vi "fric_comp_subvi.vi"(4 "Cpos":dbl, 5 "Cneg":dbl, 6 "Vpos":dbl, 7 "Vneg":dbl, 11 "Velocity":dbl) -> (3 "Numeric":dbl)   [LabVIEW 2018]
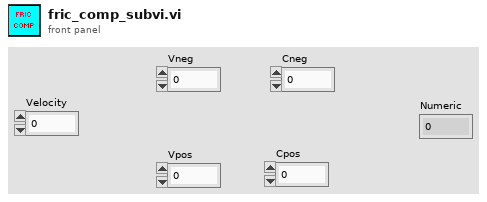
[diagram p1: front panel]
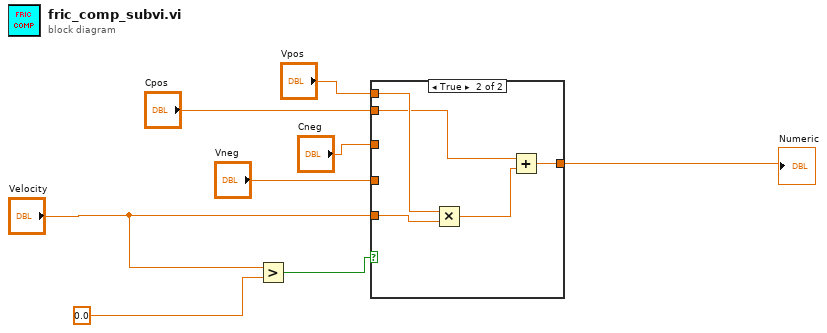
[diagram p0: block diagram]
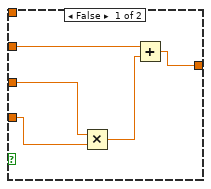
[diagram p2: hidden frame]
diagram:
  n1 = Greater?(x="Velocity", y=0.0 ("Constant")) -> (0:w1:bool)
  n2 = case shown="True" w1 {
    tunnel: "Vpos" -> [_ w18]
    tunnel: "Cpos" -> [_ w17]
    tunnel: "Velocity" -> [w12 w16]
    tunnel: [w9 w14] -> w6
    tunnel: "Vneg" -> [w13 _]
    tunnel: "Cneg" -> [w11 _]
    frame False {
      n3 = Multiply ("Multiply 2")(x=w13, y=w12) -> (x*y=w10:dbl)
      n4 = Add ("Add 2")(x=w11, y=w10) -> (x+y=w9:dbl)
    }
    frame True {
      n5 = Multiply(x=w18, y=w16) -> (x*y=w15:dbl)
      n6 = Add(x=w17, y=w15) -> (x+y=w14:dbl)
    }
  }
  "Numeric" <- w6
